vi "macro_TrajectoryConstraint_DiffVolt.vi"   [LabVIEW 2019, in "Trajectory_Library.lvlib"]
uses:
  Trajectory_Library.lvlib
types:
  T1 = typedef "Trajectory_Library.lvlib/SIMPLE_MOTOR_FF.ctl" = cluster{"Ks":dbl, "Kv":dbl, "Ka":dbl}
  T2 = typedef "Trajectory_Library.lvlib/DIFF_DRIVE_KINEMATICS.ctl" = cluster{"TrackWidth_Meters":dbl}
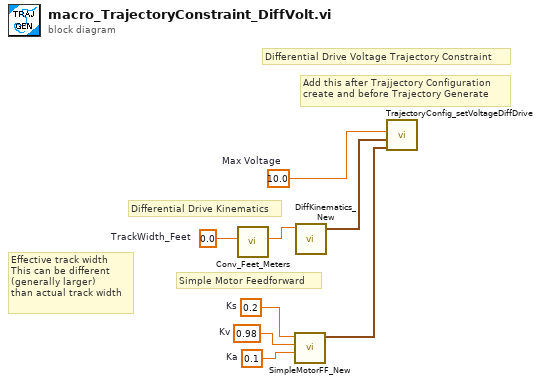
[diagram p0: block diagram]
diagram:
  w2 = 0.2  # Ks
  w3 = 0.98  # Kv
  w4 = 0.1  # Ka
  w6 = 0.0  # TrackWidth_Feet
  w8 = 10.0  # Max Voltage
  # "Differential Drive Voltage Trajectory Constraint"
  # "Add this after Trajjectory Configuration\ncreate and before Trajectory Generate"
  # "Simple Motor Feedforward"
  # "Differential Drive Kinematics"
  # "Effective track width\nThis can be different\n(generally larger)\nthan actual track width"
  n1 = call "Conv_Feet_Meters.vi"("Feet"=w6) -> ("Meters"=w7:dbl)  [unwired: 10 in]
  n2 = call "SimpleMotorFF_New.vi"("Ka"=w4, "Kv"=w3, "Ks"=w2) -> ("SIMPLE_MOTOR_FF"=w1:T1)  [unwired: 8 in]
  n3 = call "DiffKinematics_New.vi"("TrackWidth_Meters"=w7) -> ("DIFF_DRIVE_KINEMATICS"=w5:T2)  [unwired: 10 in]
  n4 = call "TrajectoryConfig_setVoltageDiffDrive.vi"("SIMPLE_MOTOR_FF"=w1, "DIFF_DRIVE_KINEMATICS"=w5, "Max Voltage"=w8) -> ()  [unwired: 8 in, 1 out]
